vi "Get Referenced Nodes.vi"(8 "error in (no error)":errorcluster, 11 "Item Ref in":T1 format="%.0x") -> (0 "error out":errorcluster, 2 "Array":T1[](array[typedef]) format="%.0x", 3 "Item Ref out":T1 format="%.0x")   [LabVIEW 2026, in "WebPage Addon System Explorer.lvlib"]
uses:
  WebPage Addon System Explorer.lvlib
  <vilib>/NI VeriStand/Custom Device API/Custom Device Item Ref.ctl
  <vilib>/NI VeriStand/Custom Device API/Get Item Property (Dependent Node Pointer).vi
  <vilib>/NI VeriStand/Custom Device API/Custom Device API.lvlib
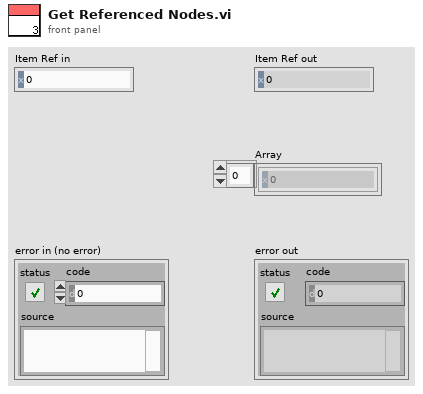
[diagram p1: front panel]
types:
  T1 = typedef "Custom Device API.lvlib/Custom Device Item Ref.ctl" = u64
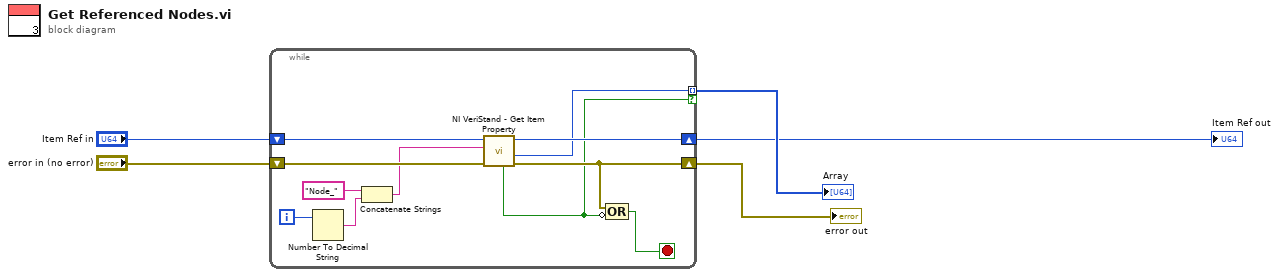
[diagram p0: block diagram]
diagram:
  n1 = while {
    shift-right: [w15] -> w3
    shift-left: "Item Ref in" -> [w16]
    shift-right: [w8] -> w4
    shift-left: "error in (no error)" -> [w14]
    tunnel: [w7] -> w5 mode=indexing if=w6
    i -> [w12]
    stop <- w9 stop-if-true
    n2 = Number To Decimal String(number=w12) -> (decimal integer string=w11:string)  [unwired: 1 in]
    n3 = Concatenate Strings("Node_", w11) -> (w10:string)
    n4 = call-poly <vilib>:"NI VeriStand - Get Item Property.vi"("error in (no error)"=w14, "Property Name"=w10, "Item Ref in"=w16) -> ("error out"=w8:errorcluster, "Dependent Node Ref"=w7:T1, "Item Ref out"=w15:T1, "Found"=w6:bool)  [unwired: 5 in]
    n5 = Compound Arithmetic op=OR(w8, invert w6) -> (w9:bool)
  }
  "Array" <- w5
  "error out" <- w4
  "Item Ref out" <- w3
